vi "InTurtleMode.vi"(9 "MaxStayForce":dbl, 10 "WindSpeed (m/s)":dbl, 11 "HindbrainEmergencySailOverrideOn":bool) -> (3 "InTurtleMode?":bool)   [LabVIEW 2013]
doc: "This VI is intended to sense the Hindbrain emergency mode and call a Midbrain emergency if the Hindbrain calls a number of emergencies in a short period of time. If the Hindbrain is frequently letting out the sails due to excessive stress, the Midbrain should put the boat in turtle mode for some medium length of time, maybe a minute or two, and determine whether to come out of turtle mode based on whether both the wind speed and stay forces are in safe bounds.\n\nThis will need some sort of relative time reference, for two reasons. First, it will be needed in order to say \"how many HB emergencies have happened in the last 5 minutes?\". Second, it will be needed in order to say \"I've called a MB emergency for 45 seconds, I'll return TRUE every time I am queried in the next 15 seconds\".\n\nEric Schneider, Jan. 2014"
panel:
  out "Array 2":timestamp[](array[timestamp])
  in  "stop":bool
  in  "Number of emergencies in given timestep\nbefore MB emergency is called":i32
  in  "Cutoff on how long HB emergencies\nshould be remembered (s)":dbl=60.0
  out "Array":timestamp[](array[timestamp])
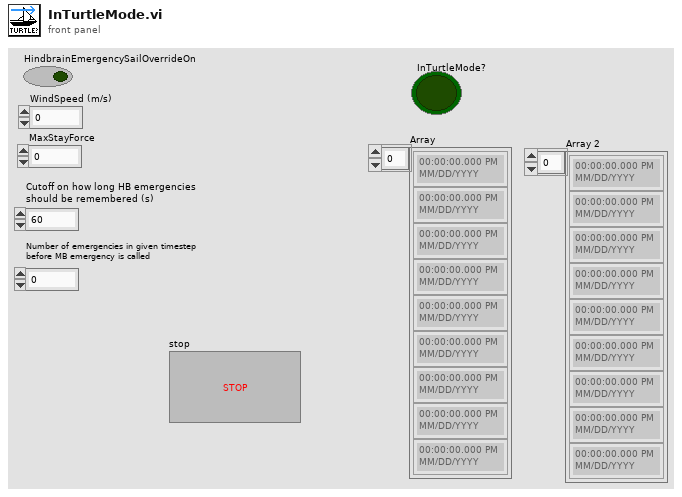
[diagram p1: front panel]
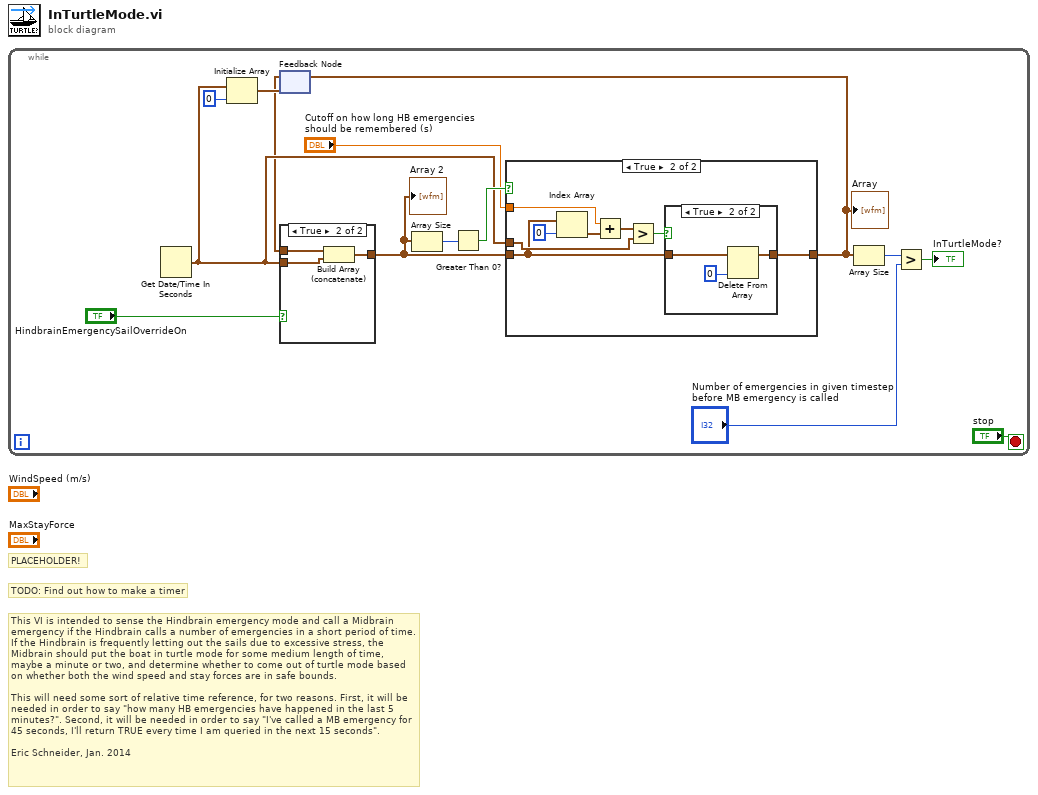
[diagram p0: block diagram]
diagram:
  # "TODO: Find out how to make a timer"
  # "PLACEHOLDER!"
  # "This VI is intended to sense the Hindbrain emergency mode and call a Midbrain emergency if the Hindbrain calls a number of emergencies in a short period of time. If the Hindbrain is frequently letting out the sails due to excessive stress, the Midbrain should put the boat in turtle mode for some medium length of time, maybe a minute or two, and determine whether to come out of turtle mode based on whether both the wind speed and stay forces are in safe bounds.\n\nThis will need some sort of relative time reference, for two reasons. First, it will be needed in order to say \"how many HB emergencies have happened in the last 5 minutes?\". Second, it will be needed in order to say \"I've called a MB emergency for 45 seconds, I'll return TRUE every time I am queried in the next 15 seconds\".\n\nEric Schneider, Jan. 2014"
  n1 = while {
    stop <- "stop" stop-if-true
    n2 = Get Date/Time In Seconds() -> (seconds since 1Jan1904=w9:timestamp)
    n3 = Initialize Array(w9, 0 ("dimension size")) -> (w2:timestamp[])
    n4 = feedback #1(w2) -> (w1:timestamp[])
    n5 = case shown="True" "HindbrainEmergencySailOverrideOn" {
      tunnel: w1 -> [w28 w31]
      tunnel: w9 -> [_ w30]
      tunnel: [w28 w29] -> w10
      frame False {
      }
      frame True {
        n6 = Build Array (concatenate)(w31, w30) -> (w29:timestamp[])
      }
    }
    "Array 2" <- w10
    n7 = Array Size(array=w10) -> (size(s)=w11:i32)
    n8 = Greater Than 0?(x=w11) -> (x > 0?=w12:bool)
    n9 = case shown="True" w12 {
      tunnel: w10 -> [w15 w20]
      tunnel: w9 -> [_ w23]
      tunnel: [w15 w19] -> w3
      tunnel: "Cutoff on how long HB emergencies\nshould be remembered (s)" -> [_ w16]
      frame False {
      }
      frame True {
        n10 = Index Array(array=w20, index=0) -> (element=w18:timestamp)
        n11 = Add(x=w16, y=w18) -> (x+y=w17:timestamp)
        n12 = Greater?(x=w17, y=w23) -> (0:w22:bool)
        n13 = case shown="True" w22 {
          tunnel: w20 -> [w24 w27]
          tunnel: [w24 w25] -> w19
          frame False {
          }
          frame True {
            n14 = Delete From Array(array=w27, index=0) -> (array with subset deleted=w25:timestamp[])  [unwired: 1 in, 1 out]
          }
        }
      }
    }
    "Array" <- w3
    n15 = feedback-in #1(w3) -> ()
    n16 = Array Size(array=w3) -> (size(s)=w7:i32)
    n17 = Greater?(x=w7, y="Number of emergencies in given timestep\nbefore MB emergency is called") -> (0:→"InTurtleMode?":bool)
  }
